vi "get Ship Textures Hotspot.vi"(11 "Ship in":refnum<class "Ship.lvclass">) -> (3 "Ship Hotspot":refnum<class "Vector 2D.lvclass">)   [LabVIEW 2021, in "Ship.lvclass"]
uses:
  Ship.lvclass
  Ship.lvclass/Ship.ctl
  Re-use Libraries/Vector 2D/Vector 2D.lvclass
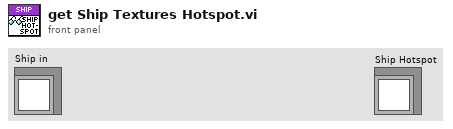
[diagram p1: front panel]
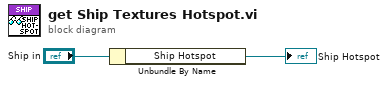
[diagram p0: block diagram]
diagram:
  n1 = Unbundle By Name("Ship in") -> ("Ship Hotspot"=→"Ship Hotspot":refnum<class "Vector 2D.lvclass">)
